vi "Big Launcher Teleop.vi"   [LabVIEW 2020]
uses:
  <vilib>/Rock Robotics/WPI/ThirdParty/Phoenix-LabVIEW/Motor Controller/Controls/CTRE_Phoenix_MotorControl_ControlMode.ctl
  Robot Global Data.vi
types:
  T1 = typedef "CTRE_Phoenix_MotorControl_ControlMode.ctl" = u16
  T2 = typedef "WPI_MotorControlDeviceRef.ctl" = cluster{"DeviceStatus":errorcluster, "Type":T3, "PWM":cluster{"PWM Channel":T4, "DeadBand":T5}, "CAN":cluster{"Device Number":u8, "SetOutput VI Ref":variant, "GetOutput VI Ref":variant, "Enable VI Ref":variant, "Disable VI Ref":variant, "Data":variant}, "Invert":bool, "DIO PWM":cluster{"PWM \"Enable\" Channel":T4, "DIOChannel":T6, "PWM Rate":dbl}}
  T3 = typedef "WPI_MotorControlType.ctl" = enum16{"PWM", "CAN", "DIO PWM"}
  T4 = typedef "FPGA_DIOPWMChannel.ctl" = enum8{"PWM 0", "PWM 1", "PWM 2", "PWM 3", "PWM 4", "PWM 5", "PWM 6", "PWM 7", "PWM 8", "PWM 9", "PWM MXP 0", "PWM MXP 1", "PWM MXP 2", "PWM MXP 3", "PWM MXP 4", "PWM MXP 5", "PWM MXP 6", "PWM MXP 7", "PWM MXP 8", "PWM MXP 9", "Invalid"}
  T5 = typedef "WPI_PWMDeadband.ctl" = cluster{"Name":string, "maxPositivePwm":i32, "minPositivePwm":i32, "centerPwm":i32, "maxNegativePwm":i32, "minNegativePwm":i32, "angularRange":u16}
  T6 = typedef "FPGA_DIOChannel.ctl" = enum8{"DIO 0", "DIO 1", "DIO 2", "DIO 3", "DIO 4", "DIO 5", "DIO 6", "DIO 7", "DIO 8", "DIO 9", "DIO MXP 0", "DIO MXP 1", "DIO MXP 2", "DIO MXP 3", "DIO MXP 4", "DIO MXP 5", "DIO MXP 6", "DIO MXP 7", "DIO MXP 8", "DIO MXP 9", "DIO MXP 10", "DIO MXP 11", "DIO MXP 12", "DIO MXP 13", "DIO MXP 14", "DIO MXP 15", "SPI Port CS1", "SPI Port CS2", "SPI Port CS3", "SPI Port MISO", "SPI Port MOSI", "Invalid"}
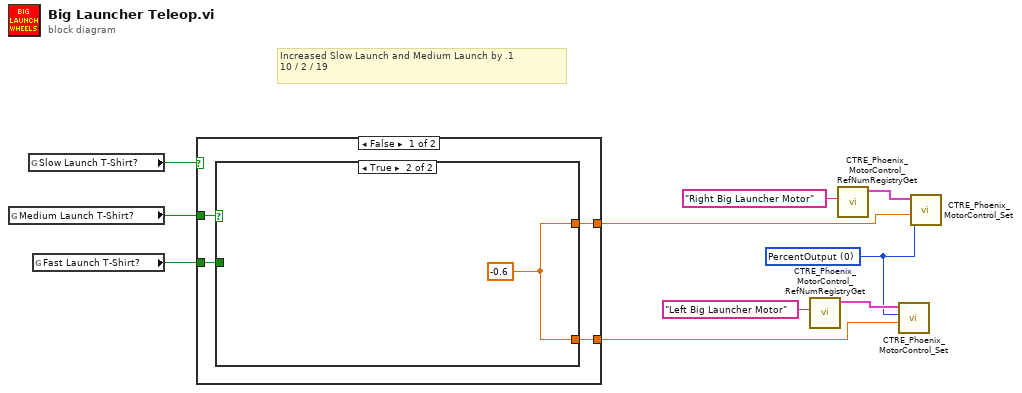
[diagram p0: block diagram]
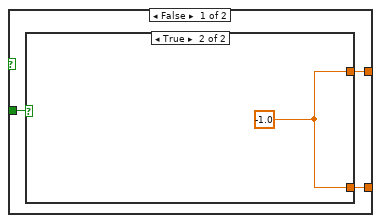
[diagram p2: hidden frame]
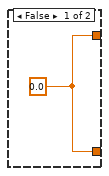
[diagram p3: hidden frame]
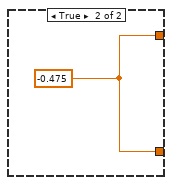
[diagram p4: hidden frame]
diagram:
  w1 = T1 0 items=["PercentOutput"=0, "Position"=1, "Velocity"=2, "Current"=3, "Follower"=5, "MotionProfile"=6, "MotionMagic"=7, "MotionProfileArc"=10, "Disabled"=15] ("Control Mode")
  # "Increased Slow Launch and Medium Launch by .1\n10 / 2 / 19"
  n1 = global read "Robot Global Data.vi" "Medium Launch T-Shirt?"() -> (w3:bool)
  n2 = global read "Robot Global Data.vi" "Slow Launch T-Shirt?"() -> (w10:bool)
  n3 = global read "Robot Global Data.vi" "Fast Launch T-Shirt?"() -> (w2:bool)
  n4 = case shown="False" w10 {
    tunnel: [w11 w21] -> w5
    tunnel: [w12 w21] -> w4
    tunnel: w3 -> [w14 _]
    tunnel: w2 -> [w13 _]
    frame False {
      n5 = case shown="True" w14 {
        tunnel: w13 -> [w17 _]
        tunnel: [w16 w20] -> w12
        tunnel: [w15 w20] -> w11
        frame False {
          n6 = case shown="True" w17 {
            tunnel: [w18 w19] -> w16
            tunnel: [w18 w19] -> w15
            frame False {
              w18 = 0.0
            }
            frame True {
              w19 = -1.0 ("Speed")
            }
          }
        }
        frame True {
          w20 = -0.6
        }
      }
    }
    frame True {
      w21 = -0.475
    }
  }
  n7 = call <vilib>:"CTRE_Phoenix_MotorControl_RefNumRegistryGet.vi"("refnum name"="Left Big Launcher Motor") -> ("PhoenixMotorControlDevRef"=w7:T2)  [unwired: 9 in, 1 out]
  n8 = call <vilib>:"CTRE_Phoenix_MotorControl_RefNumRegistryGet.vi"("refnum name"="Right Big Launcher Motor") -> ("PhoenixMotorControlDevRef"=w6:T2)  [unwired: 9 in, 1 out]
  n9 = call <vilib>:"CTRE_Phoenix_MotorControl_Set.vi"("Output"=w5, "Control Mode"=w1, "PhoenixMotorControlDevRef"=w7) -> ()  [unwired: 7 in, 2 out]
  n10 = call <vilib>:"CTRE_Phoenix_MotorControl_Set.vi"("Output"=w4, "Control Mode"=w1, "PhoenixMotorControlDevRef"=w6) -> ()  [unwired: 7 in, 2 out]
